vi "Periodic Tasks.vi"(8 "error in":errorcluster) -> ()   [LabVIEW 2013]
doc: "This VI runs in parallel to other tasks. It can contain as many user-defined periodic loops as you need. These can carry out PID or other sorts of timed response."
uses:
  <vilib>/Rock Robotics/SystemInterfaces/Utilities/FPGA_UtilitiesLED Source.ctl
  <vilib>/Rock Robotics/SystemInterfaces/Utilities/FPGA_UtilitiesLED State.ctl
  <vilib>/Rock Robotics/WPI/Compressor/WPI_CompressorGetSetRefNum.vi
  Robot Global Data.vi
panel:
  in  "Iteration for Shooter Delay":dbl
  in  "Iteration for Intake Spinner":dbl
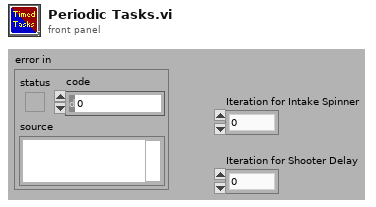
[diagram p1: front panel]
types:
  T1 = typedef "WPI_DigitalInputDevRef.ctl" = cluster{"DevStatus":errorcluster, "DIO Channel":T2, "Digital Module":T3}
  T2 = typedef "FPGA_DIOChannel.ctl" = enum8{"DIO 1", "DIO 2", "DIO 3", "DIO 4", "DIO 5", "DIO 6", "DIO 7", "DIO 8", "DIO 9", "DIO 10", "DIO 11", "DIO 12", "DIO 13", "DIO 14", "Invalid"}
  T3 = typedef "FPGA_TypedefDigitalModule.ctl" = enum16{"Digital Module 1", "Digital Module 2"}
  T4 = typedef "WPI_CompressorDevRef.ctl" = cluster{"DevStatus":errorcluster, "DigitalInputDevRef":T1, "RelayDevRef":T5}
  T5 = typedef "WPI_RelayDevRef.ctl" = cluster{"DevStatus":errorcluster, "Relay Channel":T6, "Digital Module":T3, "Relay Direction":T7}
  T6 = typedef "FPGA_DIORelayChannel.ctl" = enum8{"Relay 1", "Relay 2", "Relay 3", "Relay 4", "Relay 5", "Relay 6", "Relay 7", "Relay 8", "Invalid"}
  T7 = typedef "WPI_RelayDirection.ctl" = enum16{"Both directions", "Forward only", "Reverse only"}
  T8 = typedef "FPGA_UtilitiesLED State.ctl" = enum16{"Off", "On", "Toggle"}
  T9 = typedef "FPGA_UtilitiesLED Source.ctl" = enum16{"User LED", "FPGA LED"}
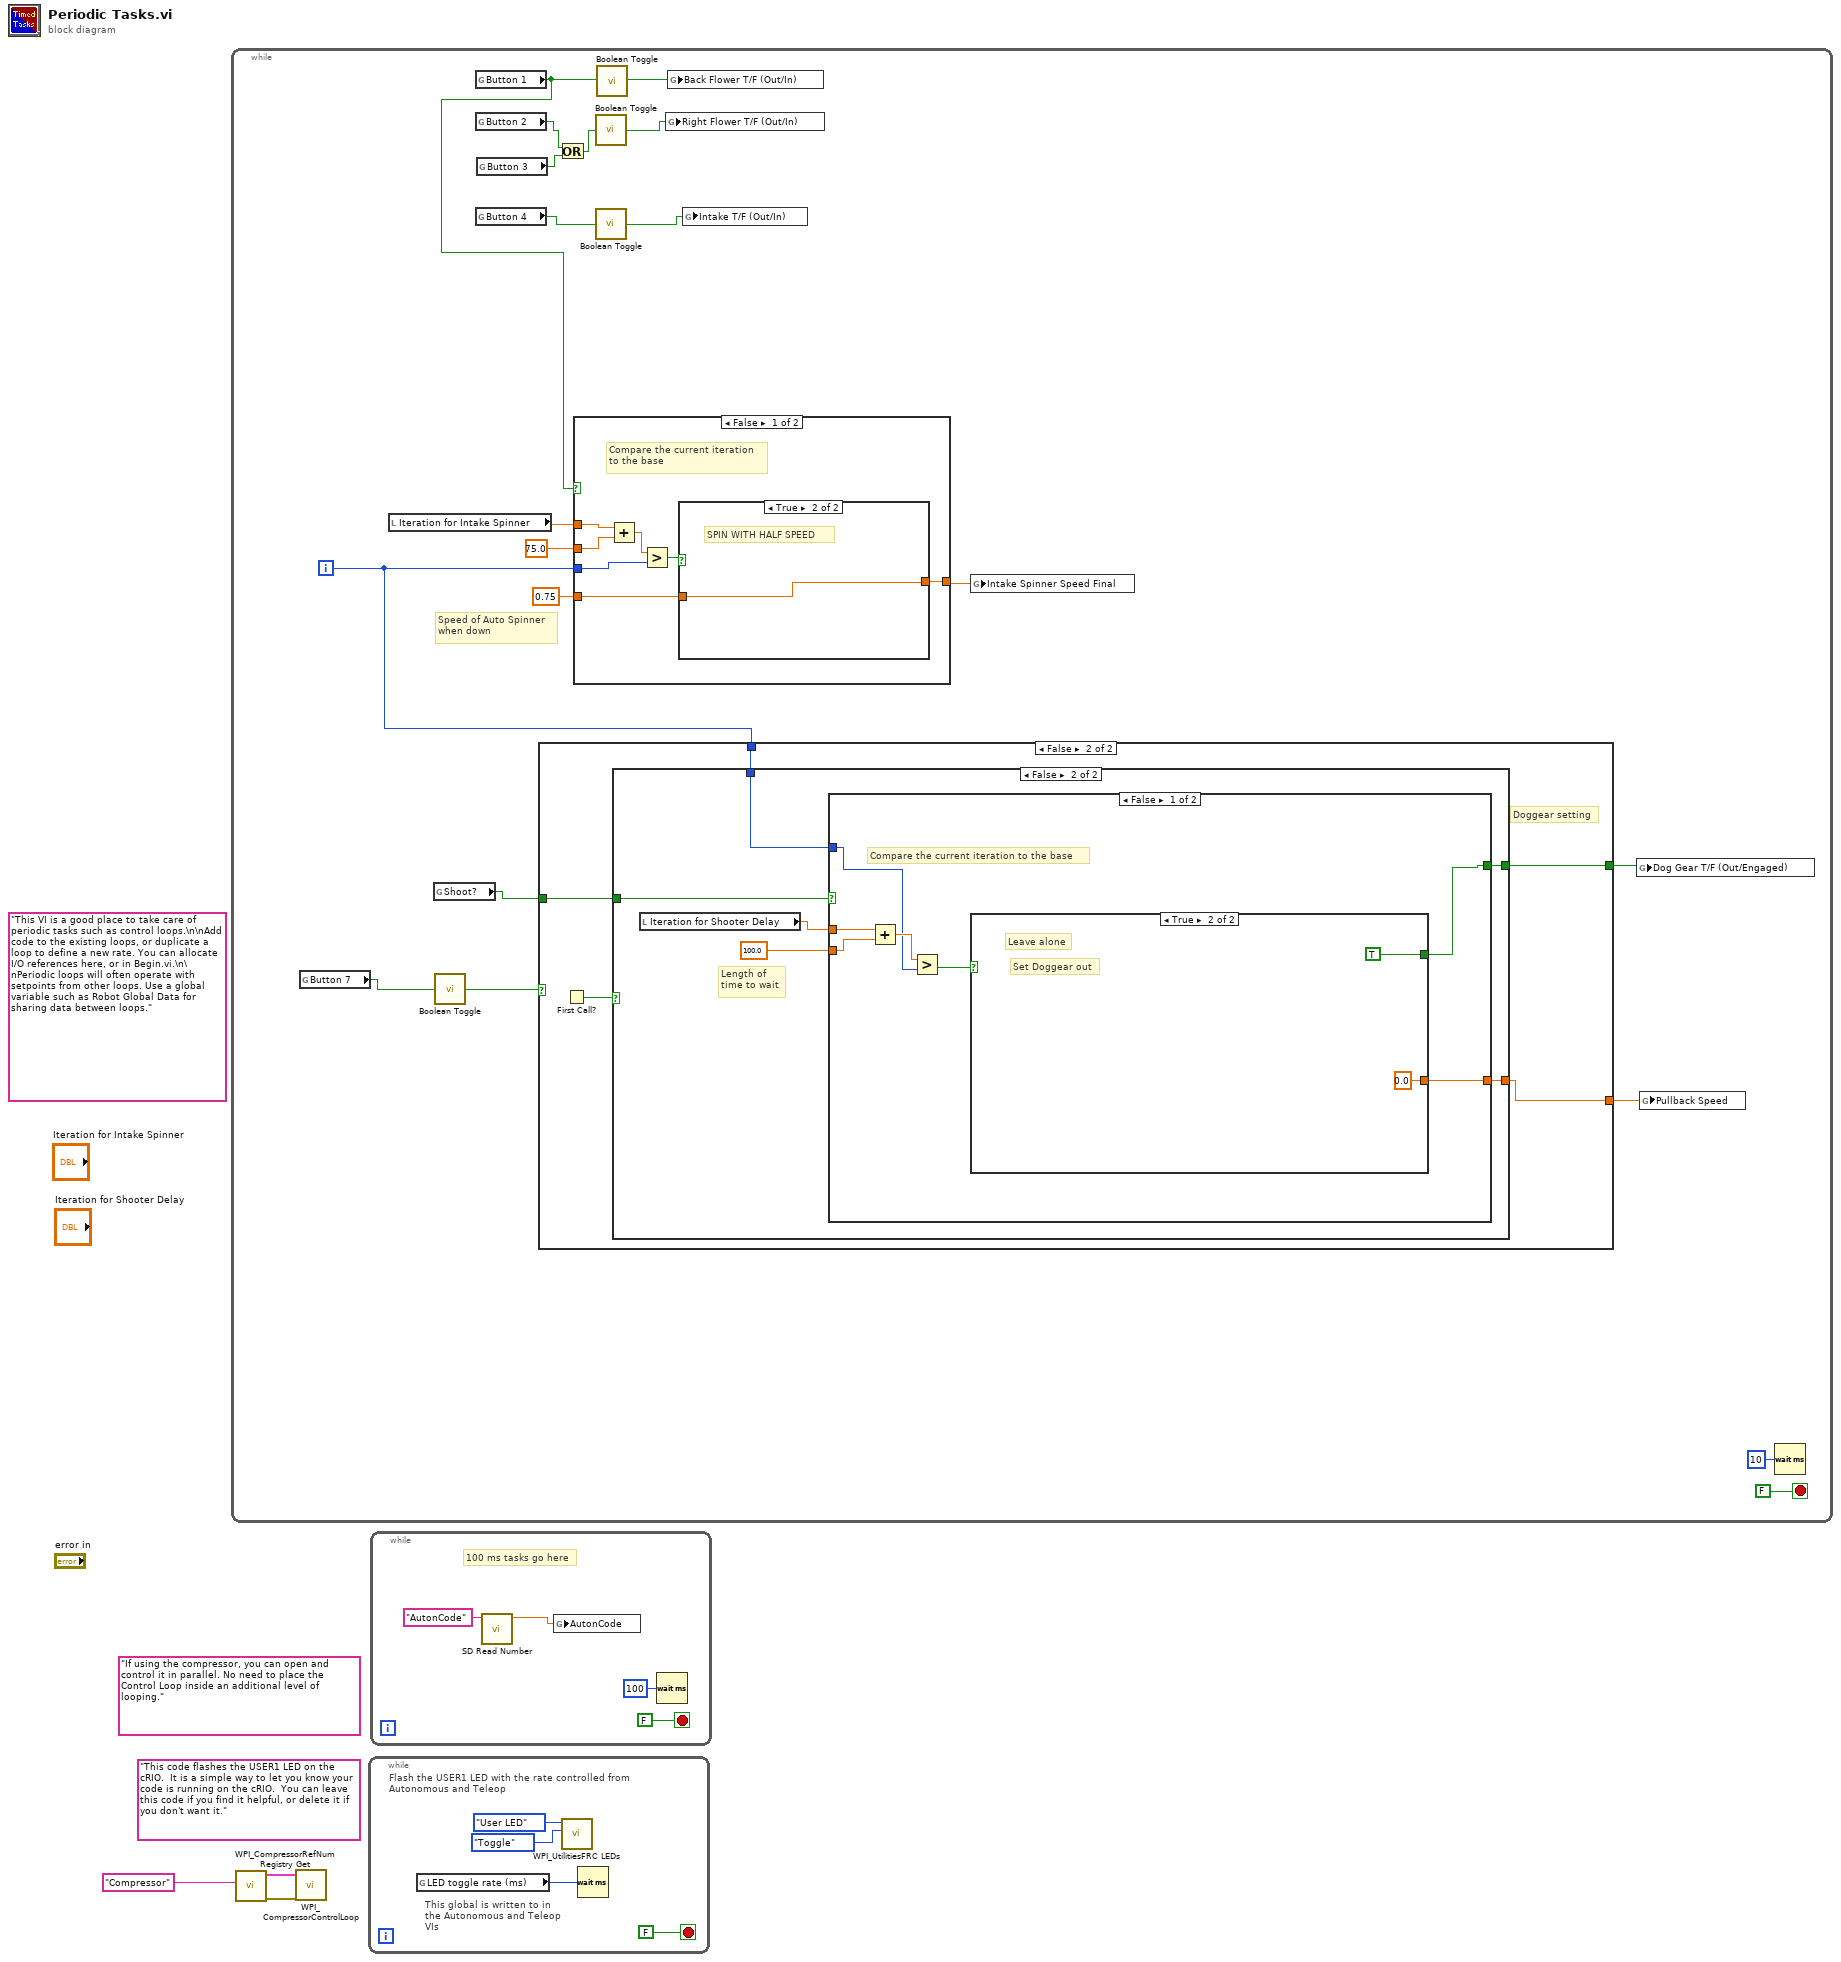
[diagram p0: block diagram]
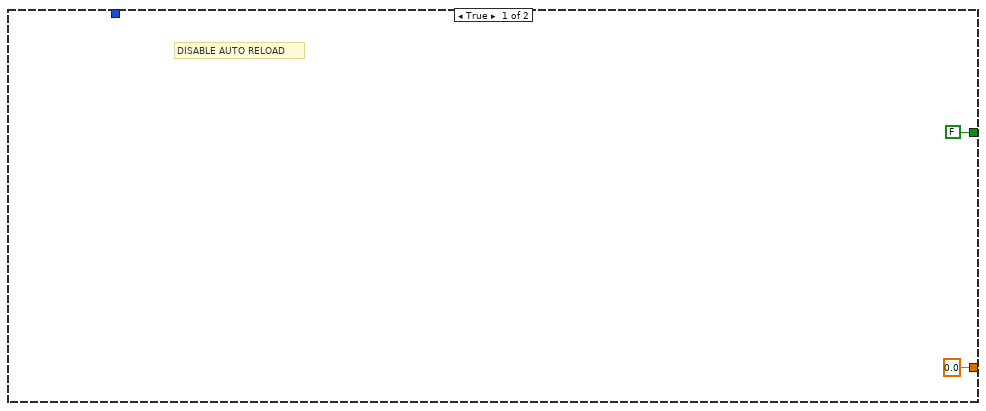
[diagram p2: hidden frame]
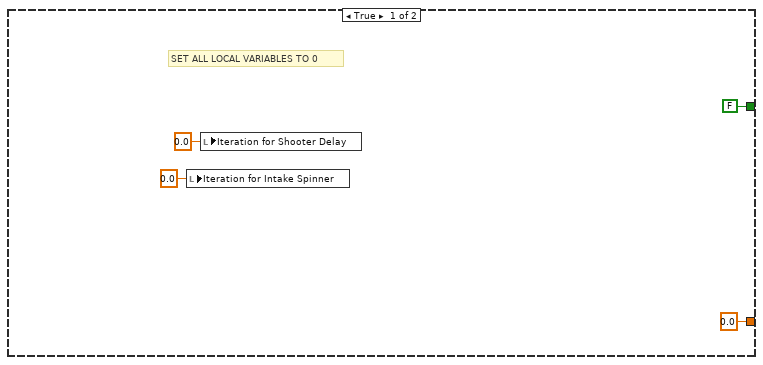
[diagram p3: hidden frame]
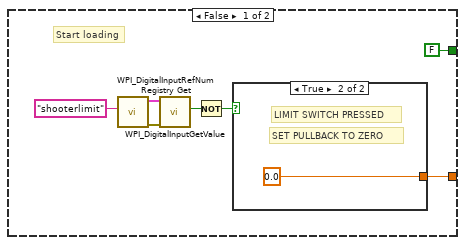
[diagram p4: hidden frame]
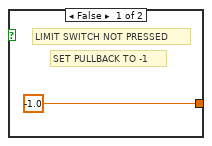
[diagram p5: hidden frame]
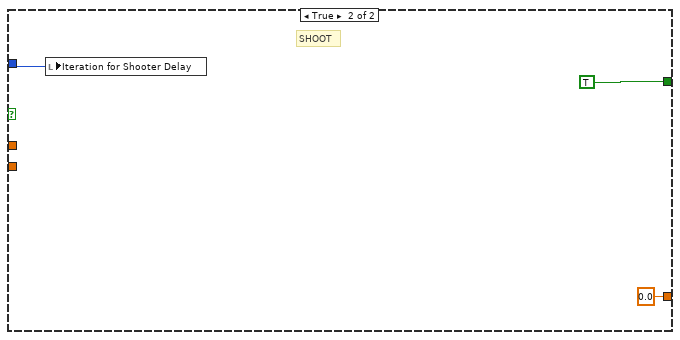
[diagram p6: hidden frame]
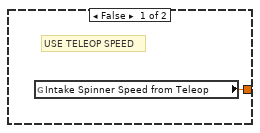
[diagram p7: hidden frame]
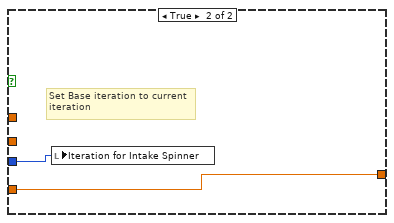
[diagram p8: hidden frame]
diagram:
  (unwired) "If using the compressor, you can open and control it in parallel. No need to place the Control Loop inside an additional level of looping."
  (unwired) "This code flashes the USER1 LED on the cRIO.  It is a simple way to let you know your code is running on the cRIO.  You can leave this code if you find it helpful, or delete it if you don't want it."
  (unwired) "This VI is a good place to take care of periodic tasks such as control loops.\n\nAdd code to the existing loops, or duplicate a loop to define a new rate. You can allocate I/O references here, or in Begin.vi.\n\nPeriodic loops will often operate with setpoints from other loops. Use a global variable such as Robot Global Data for sharing data between loops."
  n1 = while {
    i -> [w10]
    stop <- FALSE stop-if-true
    # "Speed of Auto Spinner\nwhen down"
    n2 = global read "Robot Global Data.vi" "Button 7"() -> (w8:bool)
    n3 = local read "Iteration for Intake Spinner"() -> (w15:dbl)
    n4 = global read "Robot Global Data.vi" "Shoot?"() -> (w4:bool)
    n5 = call "Boolean Toggle.vi"("Input"=w8) -> ("Output"=w7:bool)
    n6 = global read "Robot Global Data.vi" "Button 1"() -> (w12:bool)
    n7 = global read "Robot Global Data.vi" "Button 2"() -> (w17:bool)
    n8 = global read "Robot Global Data.vi" "Button 4"() -> (w13:bool)
    n9 = global read "Robot Global Data.vi" "Button 3"() -> (w18:bool)
    n10 = case shown="False" w7 {
      tunnel: w10 -> [_ w30]
      tunnel: [FALSE w29] -> w6
      tunnel: [0.0 ("Output") w28] -> w5
      tunnel: w4 -> [_ w27]
      frame True {
        # "DISABLE AUTO RELOAD"
      }
      frame False {
        # "Doggear setting"
        n11 = First Call?() -> (First Call?: T/F=w26:bool)
        n12 = case shown="False" w26 {
          tunnel: w30 -> [_ w40]
          tunnel: [FALSE w37] -> w29
          tunnel: [0.0 ("Output") w36] -> w28
          tunnel: w27 -> [_ w35]
          frame True {
            # "SET ALL LOCAL VARIABLES TO 0"
            n13 = local write "Iteration for Intake Spinner"(0.0 ("Iteration for Intake Spinner")) -> ()
            n14 = local write "Iteration for Shooter Delay"(0.0 ("Iteration for Shooter Delay")) -> ()
          }
          frame False {
            # "Length of\ntime to wait"
            n15 = local read "Iteration for Shooter Delay"() -> (w38:dbl)
            n16 = case shown="False" w35 {
              tunnel: w40 -> [w44 w61]
              tunnel: [w42 TRUE] -> w37
              tunnel: 100.0 ("y") -> [w47 _]
              tunnel: w38 -> [w46 _]
              tunnel: [w41 0.0 ("Output")] -> w36
              frame False {
                # "Compare the current iteration to the base"
                n17 = Add(x=w46, y=w47) -> (x+y=w45:dbl)
                n18 = Greater?(x=w45, y=w44) -> (0:w43:bool)
                n19 = case shown="True" w43 {
                  tunnel: [FALSE TRUE] -> w42
                  tunnel: [w49 0.0 ("Output")] -> w41
                  frame False {
                    # "Start loading"
                    n20 = call <vilib>:"WPI_DigitalInputRefNum Registry Get.vi"("refnum name"="shooterlimit") -> ("error out"=w54:errorcluster, "DigitalInputDevRef"=w53:T1)  [unwired: 9 in]
                    n21 = call <vilib>:"WPI_DigitalInputGetValue.vi"("error in (no error)"=w54, "DigitalInputDevRef"=w53) -> ("Value"=w50:bool)  [unwired: 7 in, 2 out]
                    n22 = Not(x=w50) -> (.not. x?=w51:bool)
                    n23 = case shown="True" w51 {
                      tunnel: [-1.0 ("Output") 0.0 ("Output")] -> w49
                      frame False {
                        # "LIMIT SWITCH NOT PRESSED"
                        # "SET PULLBACK TO -1"
                      }
                      frame True {
                        # "LIMIT SWITCH PRESSED"
                        # "SET PULLBACK TO ZERO"
                      }
                    }
                  }
                  frame True {
                    # "Set Doggear out"
                    # "Leave alone"
                  }
                }
              }
              frame True {
                # "SHOOT"
                n24 = local write "Iteration for Shooter Delay"(w61) -> ()
              }
            }
          }
        }
      }
    }
    n25 = Or(x=w17, y=w18) -> (x .or. y?=w16:bool)
    n26 = case shown="False" w12 {
      tunnel: w10 -> [w66 w72]
      tunnel: w15 -> [w68 _]
      tunnel: [w64 w71] -> w11
      tunnel: 0.75 ("y") -> [w63 w71]
      tunnel: 75.0 ("y") -> [w62 _]
      frame False {
        # "Compare the current iteration\nto the base"
        n27 = Add(x=w68, y=w62) -> (x+y=w67:dbl)
        n28 = Greater?(x=w67, y=w66) -> (0:w65:bool)
        n29 = case shown="True" w65 {
          tunnel: [w69 w70] -> w64
          tunnel: w63 -> [_ w70]
          frame False {
            # "USE TELEOP SPEED"
            n30 = global read "Robot Global Data.vi" "Intake Spinner Speed from Teleop"() -> (w69:dbl)
          }
          frame True {
            # "SPIN WITH HALF SPEED"
          }
        }
      }
      frame True {
        # "Set Base iteration to current\niteration"
        n31 = local write "Iteration for Intake Spinner"(w72) -> ()
      }
    }
    n32 = call "Boolean Toggle.vi"("Input"=w16) -> ("Output"=w20:bool)
    n33 = call "Boolean Toggle.vi"("Input"=w13) -> ("Output"=w21:bool)
    n34 = call "Boolean Toggle.vi"("Input"=w12) -> ("Output"=w19:bool)
    n35 = global write "Robot Global Data.vi" "Right Flower T/F (Out/In)"(w20) -> ()
    n36 = global write "Robot Global Data.vi" "Back Flower T/F (Out/In)"(w19) -> ()
    n37 = global write "Robot Global Data.vi" "Intake T/F (Out/In)"(w21) -> ()
    n38 = global write "Robot Global Data.vi" "Intake Spinner Speed Final"(w11) -> ()
    n39 = global write "Robot Global Data.vi" "Dog Gear T/F (Out/Engaged)"(w6) -> ()
    n40 = global write "Robot Global Data.vi" "Pullback Speed"(w5) -> ()
    n41 = Wait (ms)(milliseconds to wait=u32 10) -> ()  [unwired: 1 out]
  }
  n42 = call <vilib>:"WPI_CompressorRefNum Registry Get.vi"("refnum name"="Compressor") -> ("error out"=w3:errorcluster, "CompressorDevRef"=w2:T4)  [unwired: 9 in]
  n43 = call <vilib>:"WPI_CompressorControlLoop.vi"("error in (no error)"=w3, "CompressorDevRef"=w2) -> ()  [unwired: 10 in]
  n44 = while {
    stop <- FALSE stop-if-true
    # "This global is written to in the Autonomous and Teleop VIs"
    # "Flash the USER1 LED with the rate controlled from Autonomous and Teleop"
    n45 = global read "Robot Global Data.vi" "LED toggle rate (ms)"() -> (w73:u32)
    n46 = call <vilib>:"WPI_UtilitiesFRC LEDs.vi"("State"=FPGA_UtilitiesLED_State."Toggle", "LED Type"=FPGA_UtilitiesLED_Source."User LED") -> ()  [unwired: 1 in, 9 out]
    n47 = Wait (ms)(milliseconds to wait=w73) -> ()  [unwired: 1 out]
  }
  n48 = while {
    stop <- FALSE stop-if-true
    # "100 ms tasks go here"
    n49 = call <vilib>:"SD Read Number.vi"("Name"="AutonCode") -> ("Numeric"=w77:dbl)  [unwired: 8 in, 2 out]
    n50 = global write "Robot Global Data.vi" "AutonCode"(w77) -> ()
    n51 = Wait (ms)(milliseconds to wait=u32 100) -> ()  [unwired: 1 out]
  }
